vi "tb_08-nic.vi"(0 "Etude":T2, 1 "Aff ?":bool, 5 "VS":T4, 7 "ent-2D":string[][](array[string]), 9 "do-2D":string[][](array[string]), 11 "tb in ?":bool[](array[boolean])) -> (4 "Etude":T2, 6 "VS":T4, 8 "ent-2D":T1[][](array[typedef]), 10 "do-2D":string[][](array[string]), 12 "Xc":string[](array[string]), 13 "Xc-ent":T1, 14 "Xc-lib":T1, 15 "tb in ?":bool[](array[boolean]))   [LabVIEW 2010, in "lv_04.lvlib"]
uses:
  lv_04/lv_04.lvlib
  lv_04/commandes/cX.ctl
  lv_04/commandes/cSTA_varid.ctl
  lv_04/commandes/c_TDMS_ch_variable.ctl
  lv_04/commandes/c_TDMS_ch_donnees.ctl
  lv_04/commandes/c0-var-n.ctl
  lv_04/commandes/cSTA_num_do_cr.ctl
  lv_04/commandes/c02-do-num.ctl
  lv_04/commandes/c04-stat-num.ctl
  lv_04/commandes/cSTA_txt_do_cr.ctl
  lv_04/commandes/c02-do-txt.ctl
  lv_04/commandes/c04-stat-txt.ctl
  lv_04/commandes/cSTA_dist.ctl
  lv_04/commandes/c03-dist-S.ctl
  lv_04/commandes/c0-dist-xy.ctl
  lv_04/commandes/c03-dist-T.ctl
  lv_04/commandes/c03-dist-SPC.ctl
  lv_04/commandes/c_etude.ctl
  lv_02/p_5E_ch_loi.ctl
  lv_01/type format.ctl
  lv_01/lv_01.lvlib
  lv_02/lv_02.lvlib
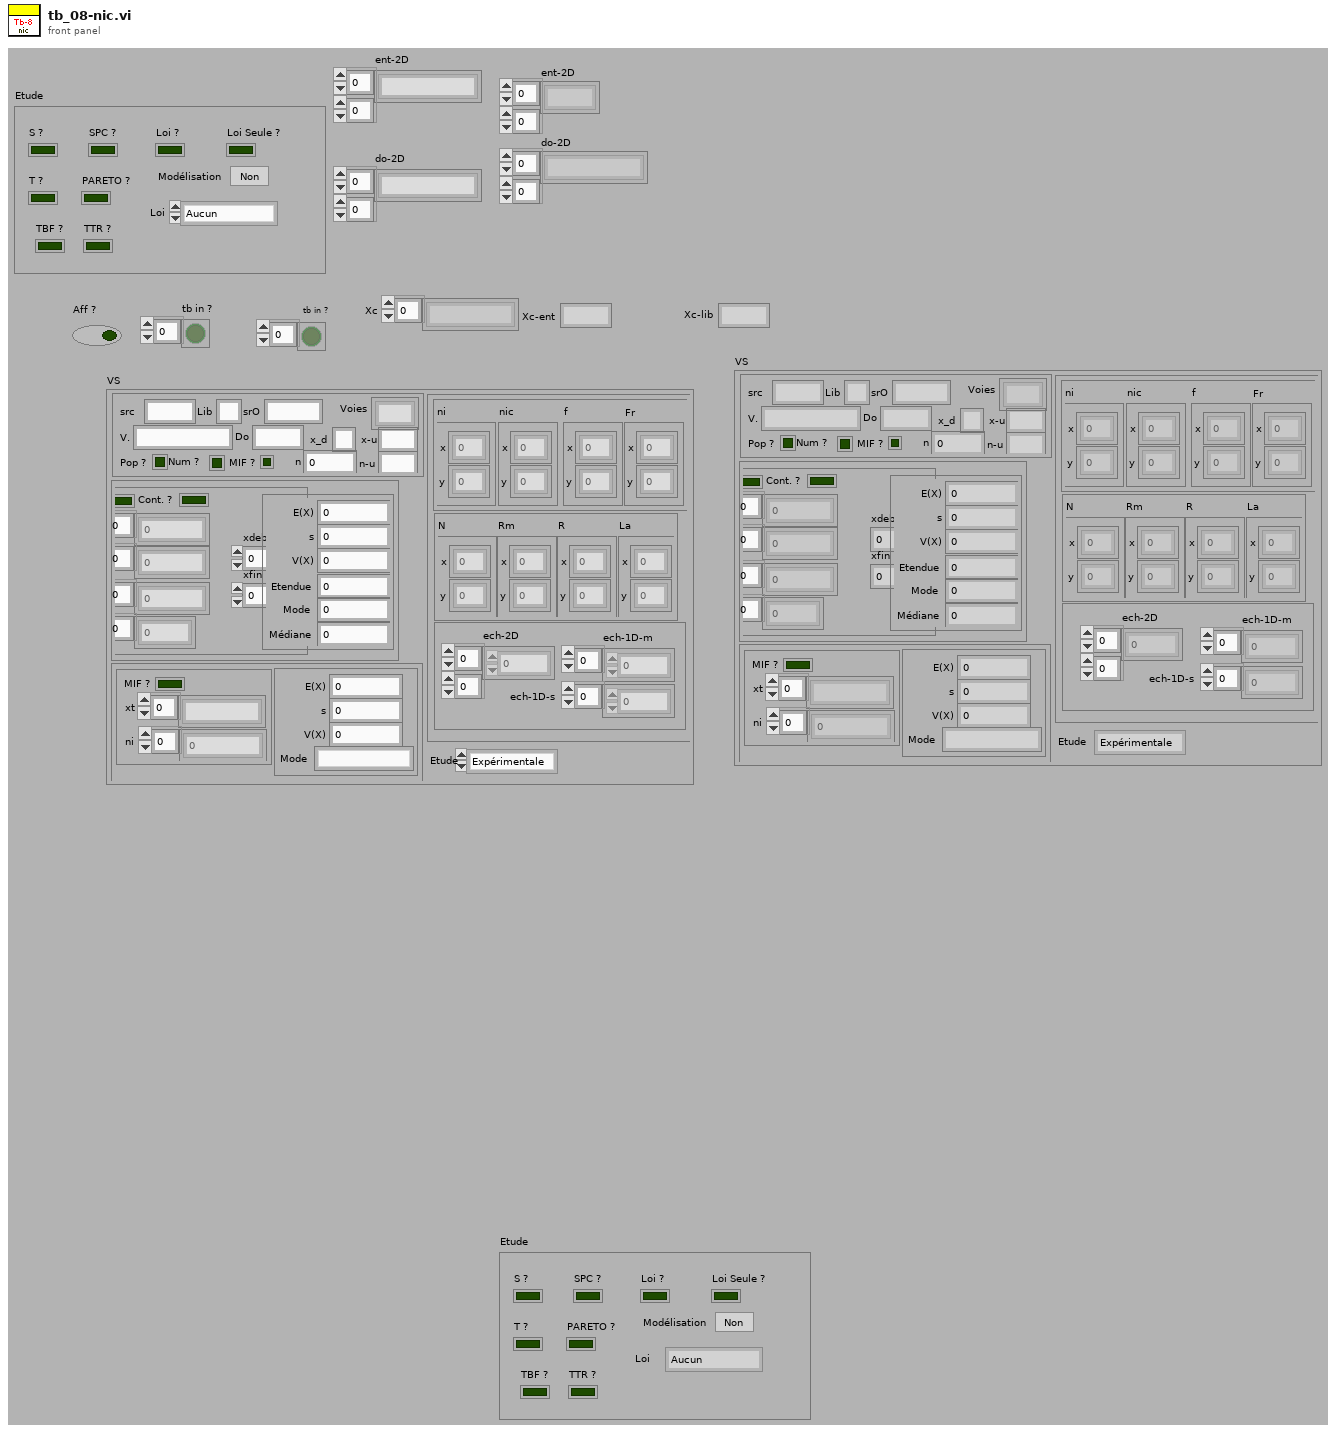
[diagram p1: front panel]
types:
  T1 = typedef "lv_04.lvlib/c_TDMS_ch_donnees.ctl" = string
  T2 = typedef "lv_04.lvlib/c_etude.ctl" = cluster{"T ?":bool, "S ?":bool, "SPC ?":bool, "PARETO ?":bool, "TBF ?":bool, "TTR ?":bool, "Loi ?":bool, "Loi Seule ?":bool, "Modélisation":bool, "Loi":T3}
  T3 = typedef "lv_02.lvlib/p_5E_ch_loi.ctl" = enum16{"Aucun", "Normale", "Aucun2", "Aucun3", "Binômial", "Poisson", "Exponentiel", "Weibull", "Rang médian"}
  T4 = typedef "lv_04.lvlib/cX.ctl" = cluster{"src":T5, "num":T8, "txt":T11, "dist":T14, "Etude":enum16{"Expérimentale", "Modèle"}}
  T5 = typedef "lv_04.lvlib/cSTA_varid.ctl" = cluster{"src":string, "Lib":string, "srO":string, "V.":T6, "Voies":string[], "Do":T1, "n":T7, "Num ?":bool, "Pop ?":bool, "x_d":string, "x-u":string, "n-u":string, "MIF ?":bool}
  T6 = typedef "lv_04.lvlib/c_TDMS_ch_variable.ctl" = string
  T7 = typedef "lv_04.lvlib/c0-var-n.ctl" = i32
  T8 = typedef "lv_04.lvlib/cSTA_num_do_cr.ctl" = cluster{"do":T9, "sta":T10}
  T9 = typedef "lv_04.lvlib/c02-do-num.ctl" = cluster{"MIF ?":bool, "Cont. ?":bool, "xi":dbl[], "xic":dbl[], "ni":u32[], "dx":dbl[], "xdeb":dbl, "xfin":dbl}
  T10 = typedef "lv_04.lvlib/c04-stat-num.ctl" = cluster{"E(X)":dbl, "s":dbl, "V(X) ":dbl, "Etendue":dbl, "Mode":dbl, "Médiane":dbl}
  T11 = typedef "lv_04.lvlib/cSTA_txt_do_cr.ctl" = cluster{"do":T12, "sta":T13}
  T12 = typedef "lv_04.lvlib/c02-do-txt.ctl" = cluster{"xt":string[], "ni":dbl[], "MIF ?":bool}
  T13 = typedef "lv_04.lvlib/c04-stat-txt.ctl" = cluster{"E(X)":dbl, "s":dbl, "V(X) ":dbl, "Mode":string}
  T14 = typedef "lv_04.lvlib/cSTA_dist.ctl" = cluster{"S":T15, "T":T17, "spc":T18}
  T15 = typedef "lv_04.lvlib/c03-dist-S.ctl" = cluster{"nic":T16, "f":T16, "Fr":T16, "ni":T16}
  T16 = typedef "lv_04.lvlib/c0-dist-xy.ctl" = cluster{"x":dbl[], "y":dbl[]}
  T17 = typedef "lv_04.lvlib/c03-dist-T.ctl" = cluster{"N":T16, "Rm":T16, "R":T16, "La":T16}
  T18 = typedef "lv_04.lvlib/c03-dist-SPC.ctl" = cluster{"ech-2D":dbl[][], "ech-1D-m":dbl[], "ech-1D-s":dbl[]}
  T19 = typedef "lv_01.lvlib/type format.ctl" = enum16{"X (dbl)", "P (Proba)", "N (entier)", "S (Scient.)"}
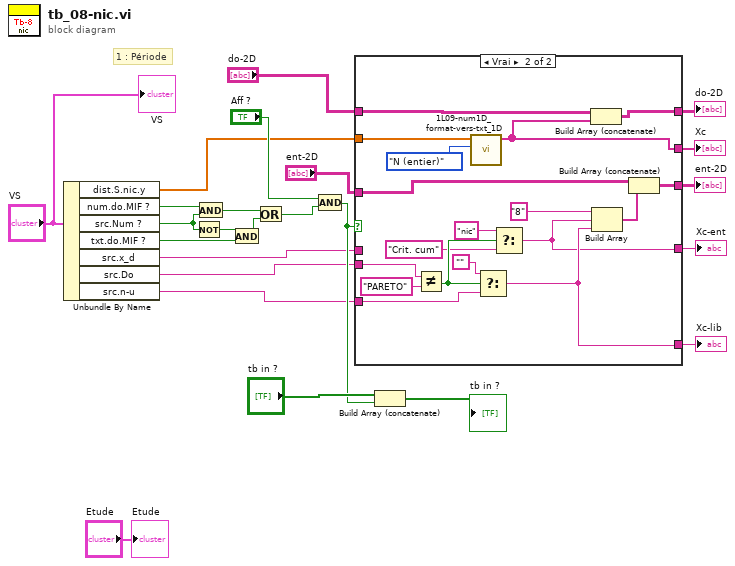
[diagram p0: block diagram]
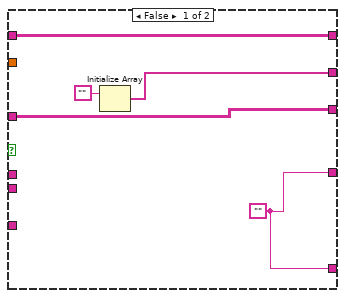
[diagram p2: hidden frame]
diagram:
  # "1 : Période"
  n1 = Unbundle By Name("VS") -> ("dist.S.nic.y"=w8:dbl[], "num.do.MIF ?"=w4:bool, "src.Num ?"=w5:bool, "txt.do.MIF ?"=w3:bool, "src.x_d"=w10:string, "src.Do"=w9:T1, "src.n-u"=w11:string)
  n2 = Not(x=w5) -> (.not. x?=w1:bool)
  n3 = And(x=w4, y=w5) -> (x .and. y?=w6:bool)
  n4 = And(x=w1, y=w3) -> (x .and. y?=w7:bool)
  n5 = Or(x=w6, y=w7) -> (x .or. y?=w2:bool)
  n6 = Compound Arithmetic op=AND("Aff ?", w2) -> (w13:bool)
  n7 = case shown="Vrai" w13 {
    tunnel: w8 -> [_ w41]
    tunnel: [w29 w39] -> w22
    tunnel: w9 -> [_ w34]
    tunnel: "do-2D" -> [w27 w47]
    tunnel: [w27 w46] -> w20
    tunnel: "ent-2D" -> [w26 w45]
    tunnel: [w26 w43] -> w18
    tunnel: [w25 w33] -> w17
    tunnel: [w25 w36] -> w16
    tunnel: w11 -> [_ w37]
    tunnel: w10 -> [_ _]
    frame False {
      w25 = ""
      n8 = Initialize Array("") -> (w29:string[])  [unwired: 1 in]
    }
    frame True {
      n9 = Not Equal?(x=w34, y=T1 "PARETO") -> (x != y?=w35:bool)
      n10 = call "1L09-num1D_format-vers-txt_1D.vi"("type"=type_format."N (entier)", "1D( num)"=w41) -> ("1D (ch)"=w39:string[])  [unwired: 7 in]
      n11 = Select(t="", s=w35, f=w37) -> (s? t:f=w36:string)
      n12 = Select(t="nic" ("cas vrai"), s=w35, f="Crit. cum") -> (s? t:f=w33:string)
      n13 = Build Array (concatenate)(w47, w39) -> (w46:string[][])
      n14 = Build Array("8", w33, w36) -> (w44:string[])
      n15 = Build Array (concatenate)(w45, w44) -> (w43:string[][])
    }
  }
  "Xc" <- w22
  "Xc-ent" <- w17
  "Xc-lib" <- w16
  "ent-2D" <- w18
  "do-2D" <- w20
  n16 = Build Array (concatenate)("tb in ?", w13) -> (→"tb in ?":bool[])
  "VS" <- "VS"
  "Etude" <- "Etude"
